vi "Values to Waveforms.vi"(11 "sensorValues":dbl[](array[numeric])) -> (1 "Pressure Transducers":waveform(dbl)[](graph), 2 "Temperature":waveform(dbl)[](graph), 3 "Load Cells":waveform(dbl)[](graph))   [LabVIEW 2022 SP3]
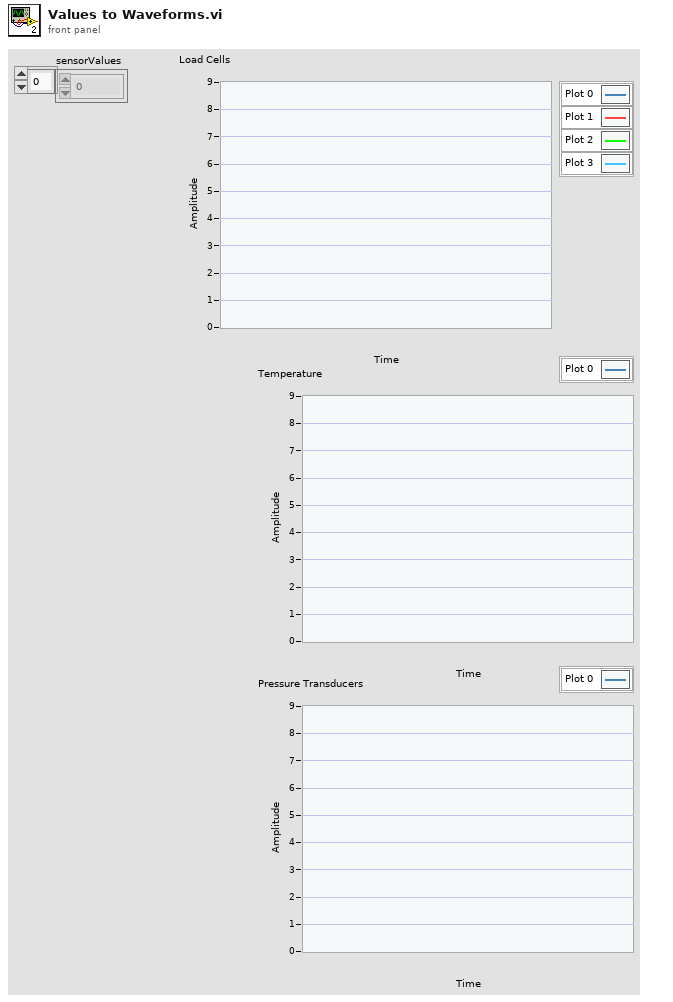
[diagram p1: front panel]
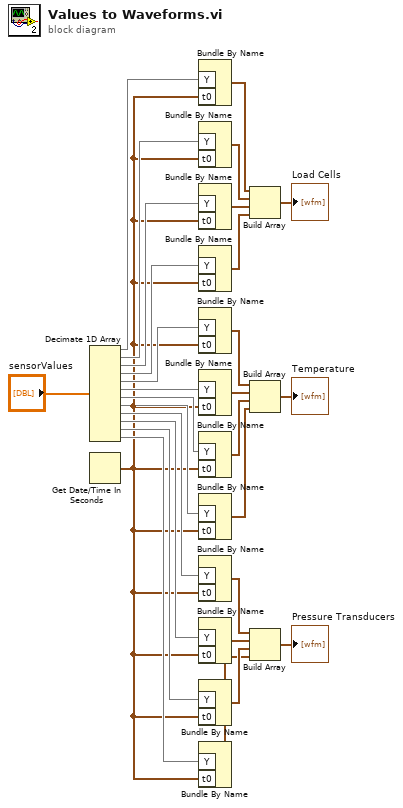
[diagram p0: block diagram]
diagram:
  n1 = Decimate 1D Array("sensorValues") -> (w24:dbl[], w23:dbl[], w22:dbl[], w21:dbl[], w9:dbl[], w8:dbl[], w7:dbl[], w6:dbl[], w5:dbl[], w4:dbl[], w3:dbl[], w2:dbl[])
  n2 = Get Date/Time In Seconds() -> (seconds since 1Jan1904=w1:timestamp)
  n3 = Bundle By Name("Y"=w24, "t0"=w1) -> (w29:waveform(dbl))  [unwired: 1 in]
  n4 = Bundle By Name("Y"=w23, "t0"=w1) -> (w28:waveform(dbl))  [unwired: 1 in]
  n5 = Bundle By Name("Y"=w22, "t0"=w1) -> (w27:waveform(dbl))  [unwired: 1 in]
  n6 = Bundle By Name("Y"=w21, "t0"=w1) -> (w26:waveform(dbl))  [unwired: 1 in]
  n7 = Bundle By Name("Y"=w9, "t0"=w1) -> (w19:waveform(dbl))  [unwired: 1 in]
  n8 = Bundle By Name("Y"=w8, "t0"=w1) -> (w18:waveform(dbl))  [unwired: 1 in]
  n9 = Bundle By Name("Y"=w7, "t0"=w1) -> (w17:waveform(dbl))  [unwired: 1 in]
  n10 = Bundle By Name("Y"=w6, "t0"=w1) -> (w16:waveform(dbl))  [unwired: 1 in]
  n11 = Bundle By Name("Y"=w5, "t0"=w1) -> (w14:waveform(dbl))  [unwired: 1 in]
  n12 = Bundle By Name("Y"=w4, "t0"=w1) -> (w13:waveform(dbl))  [unwired: 1 in]
  n13 = Bundle By Name("Y"=w3, "t0"=w1) -> (w12:waveform(dbl))  [unwired: 1 in]
  n14 = Bundle By Name("Y"=w2, "t0"=w1) -> (w11:waveform(dbl))  [unwired: 1 in]
  n15 = Build Array(w29, w28, w27, w26) -> (→"Load Cells":waveform(dbl)[])
  n16 = Build Array(w19, w18, w17, w16) -> (→"Temperature":waveform(dbl)[])
  n17 = Build Array(w14, w13, w12, w11) -> (→"Pressure Transducers":waveform(dbl)[])
